vi "Calculate X and Y pixel linear dimension.vi"(7 "Imaging Parameter.Custom":bool, 10 "Custom Size":cluster{"X":u16, "Y":u16}={"X"=1, "Y"=0} {"X" min=1 max=4096 step=1}, 11 "XY Image Resolution":T1(ring)) -> (0 "Y Px Dim (FFOV)":u16, 1 "X Px Dim (FFOV)":u16, 2 "Y Px Dim (HFOV)":u16, 3 "X Px Dim (HFOV)":u16)   [LabVIEW 2014]
doc: "This VI is used to calculate the number of linear pixels in the X and Y axis for a given image."
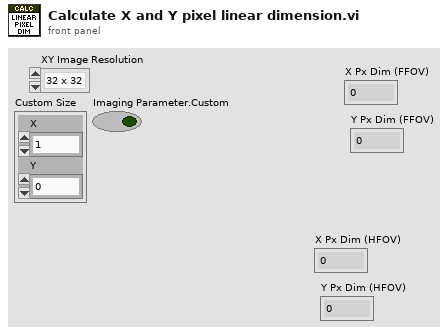
[diagram p1: front panel]
types:
  T1 = enum16{"32 x 32", "64 x 64", "128 x 128", "256 x 256", "512 x 512", "1024 x 1024", "2048 x 2048"}
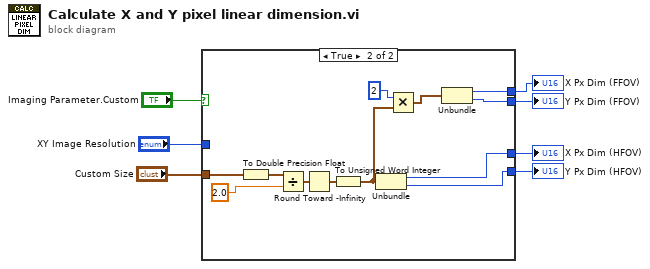
[diagram p0: block diagram]
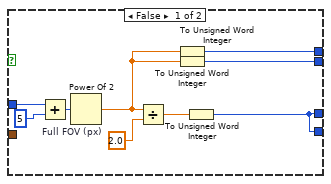
[diagram p2: hidden frame]
diagram:
  n1 = case shown="True" "Imaging Parameter.Custom" {
    tunnel: [w10 w27] -> w7
    tunnel: "XY Image Resolution" -> [w16 _]
    tunnel: "Custom Size" -> [_ w22]
    tunnel: [w10 w26] -> w3
    tunnel: [w8 w24] -> w2
    tunnel: [w9 w23] -> w1
    frame False {
      n2 = Add(x=w16, y=5) -> (x+y=w14:i32)
      n3 = Power Of 2 "Full FOV (px)"(x=w14) -> (2^x=w13:dbl)
      n4 = Divide(x=w13, y=2.0) -> (x/y=w12:dbl)
      n5 = To Unsigned Word Integer(number=w13) -> (unsigned 16bit integer=w8:u16)
      n6 = To Unsigned Word Integer(number=w13) -> (unsigned 16bit integer=w9:u16)
      n7 = To Unsigned Word Integer(number=w12) -> (unsigned 16bit integer=w10:u16)
    }
    frame True {
      n8 = To Double Precision Float(number=w22) -> (double precision float=w20:cluster{"X":dbl, "Y":dbl})
      n9 = Divide(x=w20, y=2.0) -> (x/y=w25:cluster{"X":dbl, "Y":dbl})
      n10 = Round Toward -Infinity(1:w25) -> (0:w21:cluster{"X":dbl, "Y":dbl})
      n11 = To Unsigned Word Integer(number=w21) -> (unsigned 16bit integer=w19:cluster{"X":u16, "Y":u16})
      n12 = Unbundle(w19) -> ("X"=w27:u16, "Y"=w26:u16)
      n13 = Multiply(x=u16 2, y=w19) -> (x*y=w17:cluster{"X":u16, "Y":u16})
      n14 = Unbundle(w17) -> ("X"=w24:u16, "Y"=w23:u16)
    }
  }
  "X Px Dim (HFOV)" <- w7
  "Y Px Dim (HFOV)" <- w3
  "X Px Dim (FFOV)" <- w2
  "Y Px Dim (FFOV)" <- w1
